vi "UndeferPanelUpdates.vi"(8 "error in (no error)":errorcluster, 11 "VI Reference (caller)":refnum<vi>) -> (0 "error out":errorcluster)   [LabVIEW 2014]
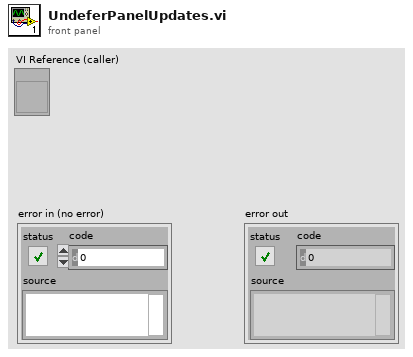
[diagram p1: front panel]
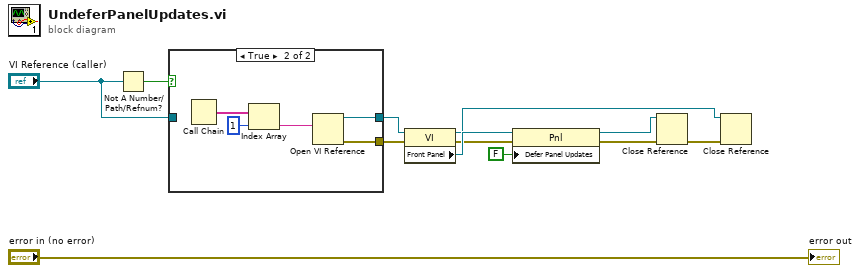
[diagram p0: block diagram]
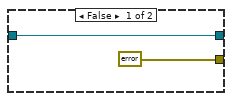
[diagram p2: hidden frame]
diagram:
  n1 = Not A Number/Path/Refnum?(number/path/refnum="VI Reference (caller)") -> (NaN/Path/Refnum?=w3:bool)
  n2 = case shown="True" w3 {
    tunnel: [w14 w17] -> w12
    tunnel: [errorcluster {"status"=FALSE, "code"=0, "source"=""} ("error out") w16] -> w4
    tunnel: "VI Reference (caller)" -> [w14 _]
    frame False {
    }
    frame True {
      n3 = Call Chain() -> (call chain=w19:string[])
      n4 = Index Array(array=w19, index=1) -> (element=w18:string)
      n5 = Open VI Reference(vi path=w18) -> (vi reference=w17:refnum<vi>, error out=w16:errorcluster)  [unwired: 5 in]
    }
  }
  n6 = property class="VI"(reference=w12, error in=w4) -> (reference out=w6:refnum<vi>, error out=w5:errorcluster, "Front Panel"=w11:refnum<vi>)
  n7 = property class="Pnl"(reference=w11, error in=w5, "Defer Panel Updates"=FALSE) -> (reference out=w8:refnum<vi>, error out=w9:errorcluster)
  n8 = Close Reference(reference=w8, error in (no error)=w9) -> (error out=w7:errorcluster)
  n9 = Close Reference(reference=w6, error in (no error)=w7) -> ()  [unwired: 1 out]
  "error out" <- "error in (no error)"
